vi "ErrorHandling.vi"(8 "Bad Command":string, 10 "Line #":i32 format="%0.0f", 11 "Script #":i32 format="%0.0f") -> (0 "Error String":string)   [LabVIEW 2018]
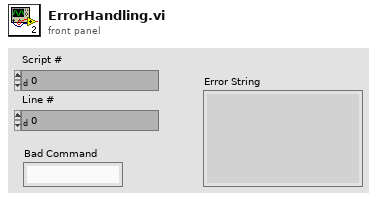
[diagram p1: front panel]
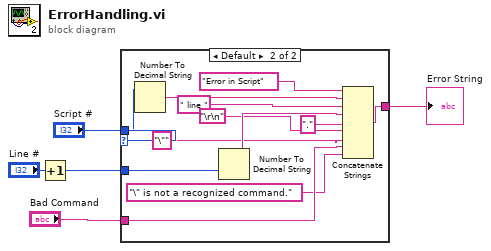
[diagram p0: block diagram]
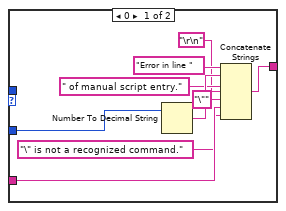
[diagram p2: hidden frame]
diagram:
  n1 = Increment(x="Line #") -> (x+1=w1:i32)
  n2 = case shown="Default" "Script #" {
    tunnel: w1 -> [w14 w25]
    tunnel: "Script #" -> [_ w24]
    tunnel: [w10 w20] -> w4
    tunnel: "Bad Command" -> [w7 w16]
    frame 0 {
      n3 = Number To Decimal String(number=w14) -> (decimal integer string=w13:string)  [unwired: 1 in]
      n4 = Concatenate Strings("Error in line ", w13, " of manual script entry." ("string"), "\r\n", "\"" ("string"), w7, "\" is not a recognized command." ("string")) -> (w10:string)
    }
    frame Default {
      n5 = Number To Decimal String(number=w24) -> (decimal integer string=w23:string)  [unwired: 1 in]
      n6 = Number To Decimal String(number=w25) -> (decimal integer string=w21:string)  [unwired: 1 in]
      n7 = Concatenate Strings("Error in Script" ("string"), w23, " line " ("string"), w21, "." ("string"), "\r\n", "\"" ("string"), w16, "\" is not a recognized command." ("string")) -> (w20:string)
    }
  }
  "Error String" <- w4
